vi "保持数据到Dat档.vi"(6 "量测数据":sgl[][](array[numeric]), 8 "选择视野":enum16{"20视野", "50视野", "100视野", "其他视野"}(ring), 9 "相机光源选项":T4, 10 "ModelEditInfo":T1 {"当前量测零件信息"."3只相机量测规格"."相机3量测规格"."上限" format="%#.4g"; "当前量测零件信息"."3只相机量测规格"."相机3量测规格"."下限" format="%#.4g"; "当前量测零件信息"."3只相机量测规格"."相机2量测规格"."上限" format="%#.4g"; "当前量测零件信息"."3只相机量测规格"."相机2量测规格"."下限" format="%#.4g"; "当前量测零件信息"."3只相机量测规格"."相机1光源2量测规格"."上限" format="%#.4g"; "当前量测零件信息"."3只相机量测规格"."相机1光源2量测规格"."下限" format="%#.4g"; "当前量测零件信息"."3只相机量测规格"."相机1光源1量测规格"."上限" format="%#.4g"; "当前量测零件信息"."3只相机量测规格"."相机1光源1量测规格"."下限" format="%#.4g"}, 11 "其他视野":dbl) -> ()   [LabVIEW 2014]
uses:
  <vilib>/Utility/file.llb/Write To Spreadsheet File (DBL).vi
  Global.vi
  Controls/SelectCamLight.ctl
  Controls/TestThreshold.ctl
  ModelEditSubVIs/CamLight.ctl
  ModelEditSubVIs/ModeEditeControl.ctl
panel:
  # "~"
  # "~"
  # "~"
  # "~"
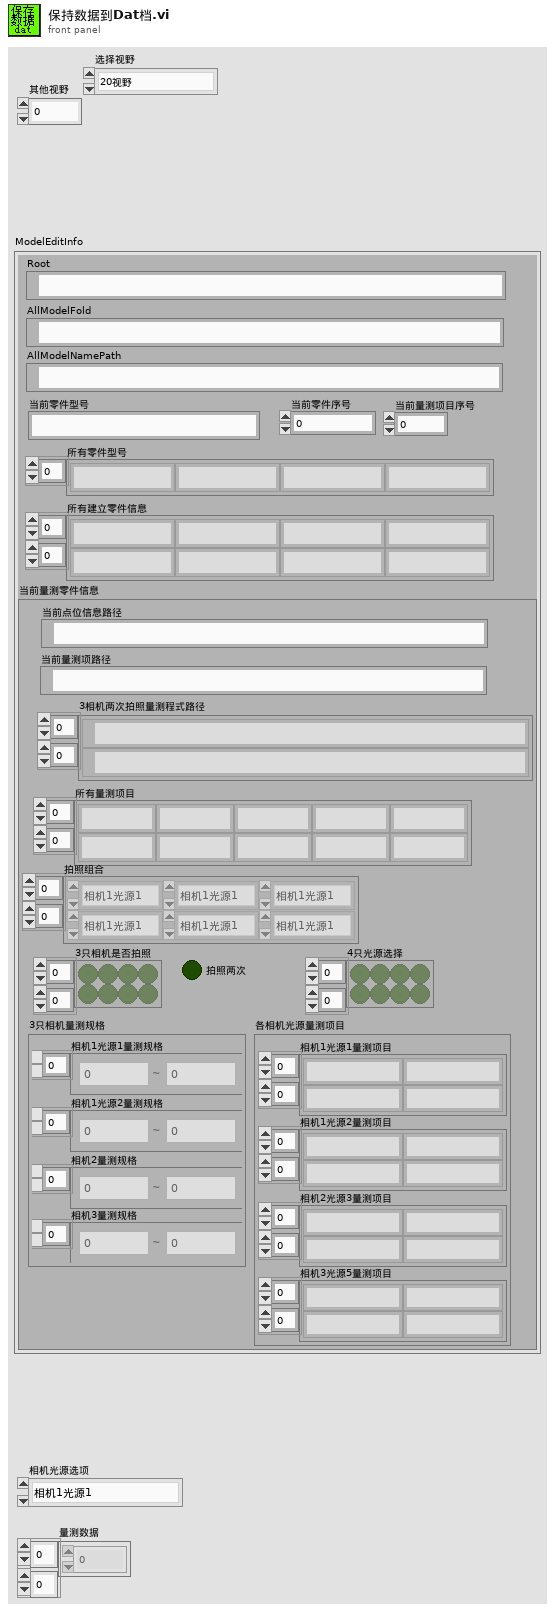
[diagram p1: front panel]
types:
  T1 = typedef "ModeEditeControl.ctl" = cluster{"Root":path, "AllModelFold":path, "AllModelNamePath":path, "所有零件型号":string[], "当前零件型号":string, "所有建立零件信息":string[][], "当前零件序号":i32, "当前量测项目序号":i32, "当前量测零件信息":cluster{"所有量测项目":string[][], "当前量测项路径":path, "3只相机量测规格":cluster{"相机1光源1量测规格":T2[], "相机1光源2量测规格":T2[], "相机2量测规格":T2[], "相机3量测规格":T2[]}, "拍照组合":T3[][], "各相机光源量测项目":cluster{"相机1光源1量测项目":string[][], "相机1光源2量测项目":string[][], "相机2光源3量测项目":string[][], "相机3光源5量测项目":string[][]}, "4只光源选择":bool[][], "3只相机是否拍照":bool[][], "拍照两次":bool, "3相机两次拍照量测程式路径":path[][], "当前点位信息路径":path}}
  T2 = typedef "TestThreshold.ctl" = cluster{"下限":dbl, "上限":dbl}
  T3 = typedef "CamLight.ctl" = enum16{"相机1光源1", "相机1光源2", "相机2光源", "相机3光源", "None"}
  T4 = typedef "SelectCamLight.ctl" = enum16{"相机1光源1", "相机1光源2", "相机2光源3", "相机2光源4", "相机3光源5", "相机3光源6"}
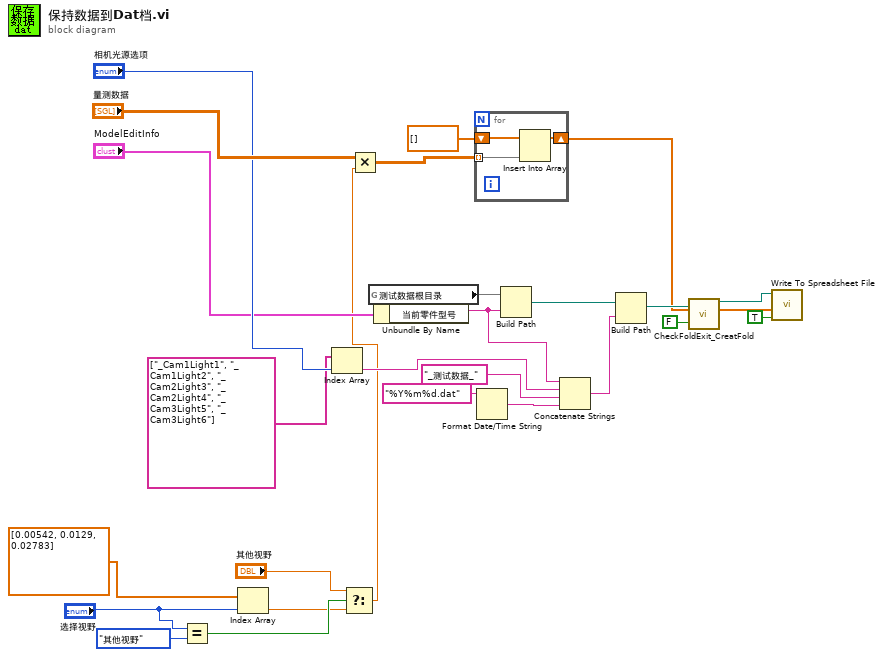
[diagram p0: block diagram]
diagram:
  n1 = Equal?(x="选择视野", y=enum16{"20视野", "50视野", "100视野", "其他视野"}."其他视野") -> (x = y?=w4:bool)
  n2 = Index Array(array=dbl[] [0.00542, 0.0129, 0.02783], index="选择视野") -> (element=w2:dbl)
  n3 = Index Array(array=string[] ["_Cam1Light1", "_Cam1Light2", "_Cam2Light3", "_Cam2Light4", "_Cam3Light5", "_Cam3Light6"], index="相机光源选项") -> (element=w19:string)
  n4 = Select(t="其他视野", s=w4, f=w2) -> (s? t:f=w1:dbl)
  n5 = Multiply(x="量测数据", y=w1) -> (x*y=w26:dbl[][])
  n6 = global read "Global.vi" "测试数据根目录"() -> (w11)
  n7 = Unbundle By Name("ModelEditInfo") -> ("当前零件型号"=w20:string)
  n8 = for {
    tunnel: w26 -> [w27] mode=indexing
    shift-right: [w28] -> w9
    shift-left: dbl[] [] -> [w29]
    n9 = Insert Into Array(array=w29, new element=w27) -> (w28:dbl[])  [unwired: 1 in]
  }
  n10 = Format Date/Time String(time format string (%c)="%Y%m%d.dat" ("时间格式字符串(%c)")) -> (date/time string=w13:string)  [unwired: 2 in]
  n11 = Build Path(base path=w11, name or relative path=w20) -> (appended path=w15:path)
  n12 = Concatenate Strings(w20, w19, "_测试数据_" ("名称或相对路径"), w13) -> (w16:string)
  n13 = Build Path(base path=w15, name or relative path=w16) -> (appended path=w23:path)
  n14 = call "CheckFoldExit_CreatFold.vi"("path in"=w23, "FoldOrFile¡H"=FALSE) -> ("File out"=w24:path)  [unwired: 2 out]
  n15 = call-poly <vilib>:"Write To Spreadsheet File.vi"("append to file? (new file:F)"=TRUE, "1D data"=w9, "file path (dialog if empty)"=w24) -> ()  [unwired: 5 in, 1 out]
